vi "AutoJump.vi"(6 "Current Index":i32, 10 "Goto":i32, 11 "Type":i32) -> (1 "Done?":bool, 4 "New Index":i32)   [LabVIEW 2014]
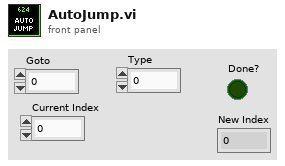
[diagram p1: front panel]
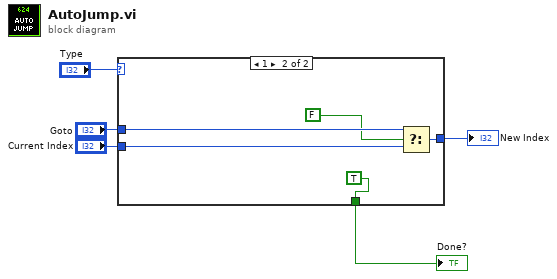
[diagram p0: block diagram]
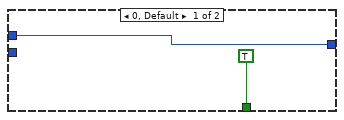
[diagram p2: hidden frame]
diagram:
  n1 = case shown="1" "Type" {
    tunnel: [w7 w10] -> w4
    tunnel: "Goto" -> [w7 w11]
    tunnel: [TRUE TRUE] -> w2
    tunnel: "Current Index" -> [_ w12]
    frame 0, Default {
    }
    frame 1 {
      n2 = Select(t=w11, s=FALSE, f=w12) -> (s? t:f=w10:i32)
    }
  }
  "Done?" <- w2
  "New Index" <- w4
